vi "fpga_input.vi"(7 "ai gain":T1) -> (3 "ai":T1)   [LabVIEW 2021]
doc: "Get input values from AO.\n\nThe input values are converted with \"ai gain\" (input = AI * ai gain)."
uses:
  fpga_dtype_sgl_8ch.ctl
  <vilib>/rvi/eio/common/nirviEmuTemplateMethod_errors.vi
  <vilib>/eio/EIONode/EIONode.xnode
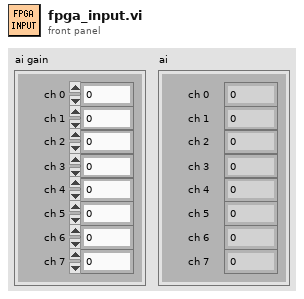
[diagram p1: front panel]
types:
  T1 = typedef "fpga_dtype_sgl_8ch.ctl" = cluster{"ch 0":sgl, "ch 1":sgl, "ch 2":sgl, "ch 3":sgl, "ch 4":sgl, "ch 5":sgl, "ch 6":sgl, "ch 7":sgl}
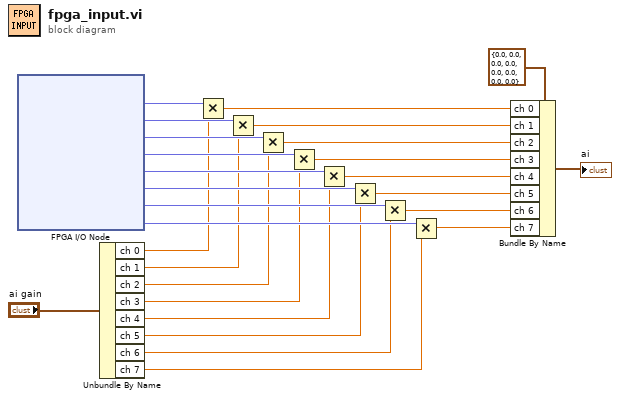
[diagram p0: block diagram]
diagram:
  n1 = xnode "FPGA I/O Node"() -> ("Connector0/AI0"=w27:fxp<+/-,27,5>, "Connector0/AI1"=w25:fxp<+/-,27,5>, "Connector0/AI2"=w24:fxp<+/-,27,5>, "Connector0/AI3"=w23:fxp<+/-,27,5>, "Connector0/AI4"=w22:fxp<+/-,27,5>, "Connector0/AI5"=w21:fxp<+/-,27,5>, "Connector0/AI6"=w20:fxp<+/-,27,5>, "Connector0/AI7"=w26:fxp<+/-,27,5>)  [unwired: 8 in, 8 out]
  n2 = Unbundle By Name("ai gain") -> ("ch 0"=w18:sgl, "ch 1"=w17:sgl, "ch 2"=w16:sgl, "ch 3"=w15:sgl, "ch 4"=w14:sgl, "ch 5"=w13:sgl, "ch 6"=w12:sgl, "ch 7"=w11:sgl)
  n3 = Multiply(x=w27, y=w18) -> (x*y=w9:sgl)
  n4 = Multiply(x=w25, y=w17) -> (x*y=w8:sgl)
  n5 = Multiply(x=w24, y=w16) -> (x*y=w7:sgl)
  n6 = Multiply(x=w23, y=w15) -> (x*y=w6:sgl)
  n7 = Multiply(x=w22, y=w14) -> (x*y=w5:sgl)
  n8 = Multiply(x=w21, y=w13) -> (x*y=w4:sgl)
  n9 = Multiply(x=w20, y=w12) -> (x*y=w3:sgl)
  n10 = Multiply(x=w26, y=w11) -> (x*y=w2:sgl)
  n11 = Bundle By Name(cluster=T1 {"ch 0"=0.0, "ch 1"=0.0, "ch 2"=0.0, "ch 3"=0.0, "ch 4"=0.0, "ch 5"=0.0, "ch 6"=0.0, "ch 7"=0.0} ("sgl 8ch"), "ch 0"=w9, "ch 1"=w8, "ch 2"=w7, "ch 3"=w6, "ch 4"=w5, "ch 5"=w4, "ch 6"=w3, "ch 7"=w2) -> (→"ai":T1)
